vi "质控启动参数选择对话框.vi"(6 "CODCr":bool, 8 "CODMn":bool, 9 "总氮":bool, 10 "总磷":bool, 11 "氨氮":bool) -> (1 "取消启动":bool, 2 "确定启动":bool, 3 "启动模块":T1)   [LabVIEW 2016, in "质控单元.lvlib"]
uses:
  <vilib>/Utility/miscctls.llb/LVPointTypeDef.ctl
panel:
  in  "CODCr":bool
  in  "总氮":bool
  in  "确定":bool
  in  "CODMn":bool
  in  "总磷":bool
  in  "取消":bool
  in  "氨氮":bool
  # "请选择加标回收模块"
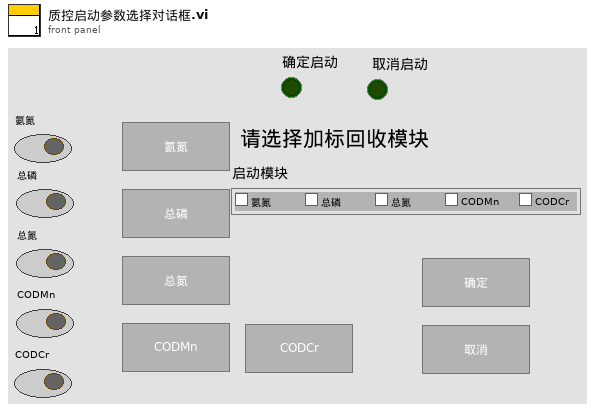
[diagram p1: front panel]
types:
  T1 = cluster{"氨氮":bool, "总磷":bool, "总氮":bool, "CODMn":bool, "CODCr":bool}
  T2 = typedef "LVPointTypeDef.ctl" = cluster{"Horizontal":i16, "Vertical":i16}
  T3 = enum8{"Enabled", "Disabled", "Disabled and Grayed Out"}
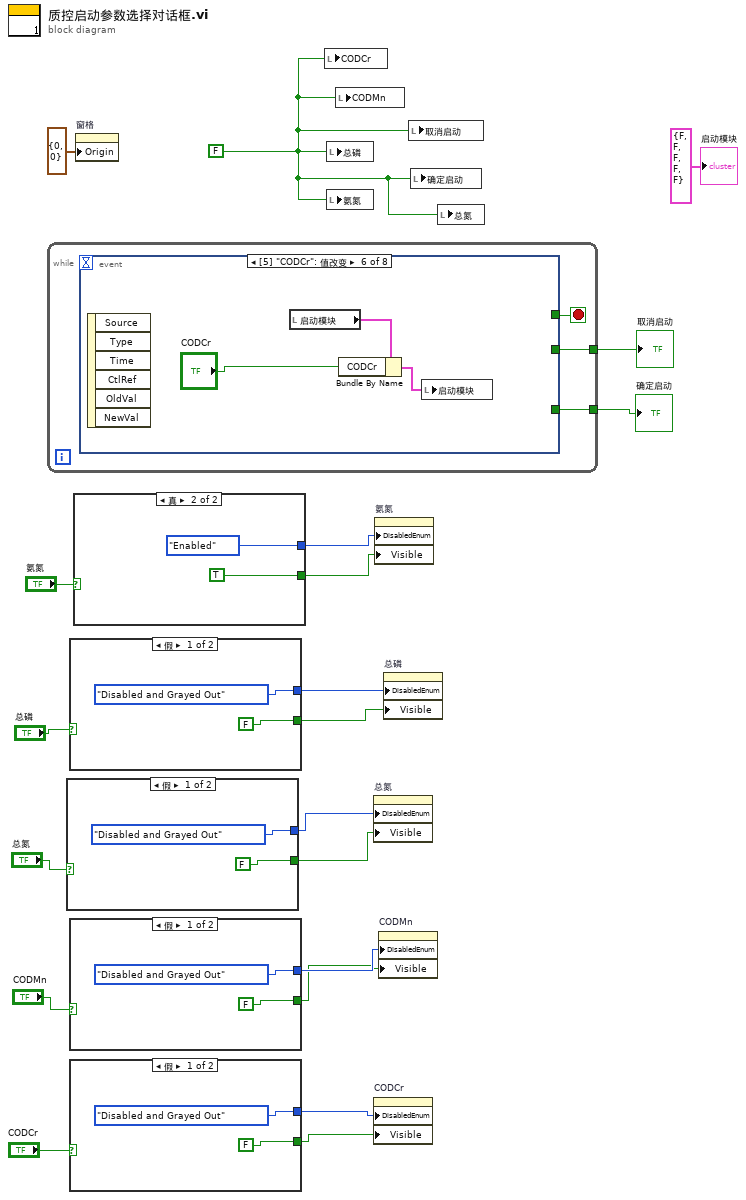
[diagram p0: block diagram]
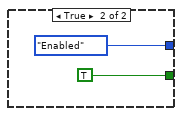
[diagram p2: hidden frame]
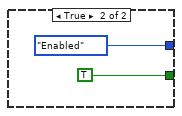
[diagram p3: hidden frame]
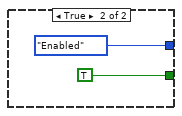
[diagram p4: hidden frame]
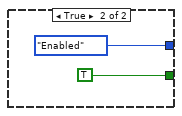
[diagram p5: hidden frame]
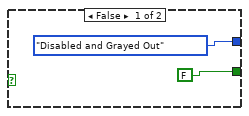
[diagram p6: hidden frame]
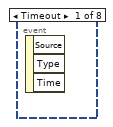
[diagram p7: hidden frame]
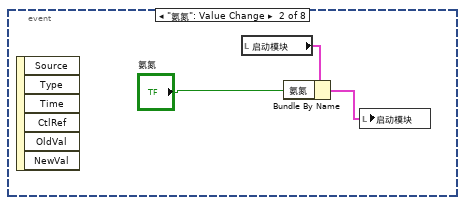
[diagram p8: hidden frame]
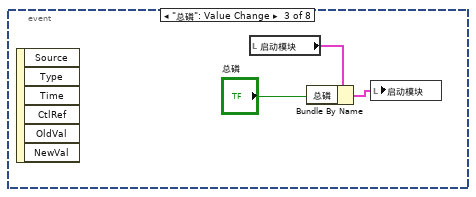
[diagram p9: hidden frame]
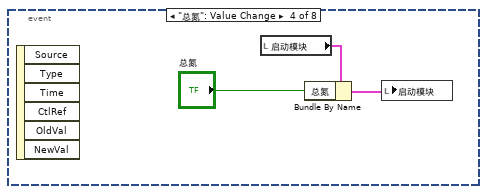
[diagram p10: hidden frame]
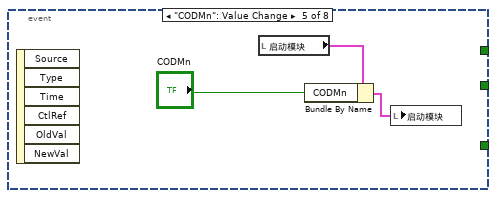
[diagram p11: hidden frame]
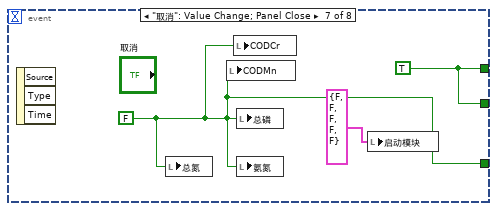
[diagram p12: hidden frame]
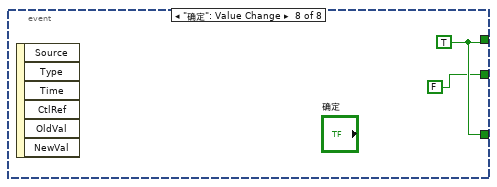
[diagram p13: hidden frame]
diagram:
  w5 = FALSE ("确定")
  n1 = while {
    tunnel: [w22] -> w20
    tunnel: [w21] -> w19
    stop <- w23 stop-if-true
    n2 = event shown="[5] \"CODCr\": 值改变" {
      selector: _ -> [_ _ _ _ _ _ _ _]
      dyn-events: _ -> [_ _ _ _ _ _ _ _]
      timeout: _ -> [_ _ _ _ _ _ _ _]
      tunnel: [_ _ _ _ _ _ w41 w43] -> w23
      tunnel: [_ _ _ _ _ _ w40 w43] -> w22
      tunnel: [_ _ _ _ _ _ w41 FALSE ("确定")] -> w21
      event Timeout {
        n3 = event-data() -> ()  [unwired: 1 in, 3 out]
      }
      event "氨氮": Value Change {
        n4 = event-data() -> ()  [unwired: 1 in, 6 out]
        n5 = local read "启动模块"() -> (w25:T1)
        n6 = Bundle By Name(cluster=w25, "氨氮"="氨氮") -> (w24:T1)
        n7 = local write "启动模块"(w24) -> ()
      }
      event "总磷": Value Change {
        n8 = event-data() -> ()  [unwired: 1 in, 6 out]
        n9 = local read "启动模块"() -> (w28:T1)
        n10 = Bundle By Name(cluster=w28, "总磷"="总磷") -> (w27:T1)
        n11 = local write "启动模块"(w27) -> ()
      }
      event "总氮": Value Change {
        n12 = event-data() -> ()  [unwired: 1 in, 6 out]
        n13 = local read "启动模块"() -> (w31:T1)
        n14 = Bundle By Name(cluster=w31, "总氮"="总氮") -> (w30:T1)
        n15 = local write "启动模块"(w30) -> ()
      }
      event "CODMn": Value Change {
        n16 = event-data() -> ()  [unwired: 1 in, 6 out]
        n17 = local read "启动模块"() -> (w34:T1)
        n18 = Bundle By Name(cluster=w34, "CODMn"="CODMn") -> (w33:T1)
        n19 = local write "启动模块"(w33) -> ()
      }
      event "CODCr": Value Change {
        n20 = event-data() -> ()  [unwired: 1 in, 6 out]
        n21 = local read "启动模块"() -> (w38:T1)
        n22 = Bundle By Name(cluster=w38, "CODCr"="CODCr") -> (w37:T1)
        n23 = local write "启动模块"(w37) -> ()
      }
      event "取消": Value Change; Panel Close {
        w40 = FALSE ("确定")
        w41 = TRUE ("确定")
        n24 = event-data() -> ()  [unwired: 1 in, 3 out]
        n25 = local write "总氮"(w40) -> ()
        n26 = local write "CODMn"(w40) -> ()
        n27 = local write "CODCr"(w40) -> ()
        n28 = local write "总磷"(w40) -> ()
        n29 = local write "氨氮"(w40) -> ()
        n30 = local write "启动模块"(T1 {"氨氮"=FALSE, "总磷"=FALSE, "总氮"=FALSE, "CODMn"=FALSE, "CODCr"=FALSE} ("启动模块")) -> ()
      }
      event "确定": Value Change {
        w43 = TRUE ("确定")
        n31 = event-data() -> ()  [unwired: 1 in, 6 out]
      }
    }
  }
  "确定启动" <- w20
  "取消启动" <- w19
  n32 = case shown="假" "总氮" {
    tunnel: [T3."Disabled and Grayed Out" ("禁用") T3."Enabled" ("禁用")] -> w10
    tunnel: [FALSE ("可见") TRUE ("可见")] -> w9
    frame False {
    }
    frame True {
    }
  }
  n33 = case shown="假" "总磷" {
    tunnel: [T3."Disabled and Grayed Out" ("禁用") T3."Enabled" ("禁用")] -> w12
    tunnel: [FALSE ("可见") TRUE ("可见")] -> w11
    frame False {
    }
    frame True {
    }
  }
  n34 = case shown="假" "CODMn" {
    tunnel: [T3."Disabled and Grayed Out" ("禁用") T3."Enabled" ("禁用")] -> w8
    tunnel: [FALSE ("可见") TRUE ("可见")] -> w7
    frame False {
    }
    frame True {
    }
  }
  n35 = case shown="假" "CODCr" {
    tunnel: [T3."Disabled and Grayed Out" ("禁用") T3."Enabled" ("禁用")] -> w2
    tunnel: [FALSE ("可见") TRUE ("可见")] -> w1
    frame False {
    }
    frame True {
    }
  }
  n36 = case shown="真" "氨氮" {
    tunnel: [T3."Disabled and Grayed Out" ("禁用") T3."Enabled" ("禁用")] -> w14
    tunnel: [FALSE ("可见") TRUE ("可见")] -> w13
    frame False {
    }
    frame True {
    }
  }
  n37 = property on="窗格" class="Pane"("Origin"=T2 {"Horizontal"=0, "Vertical"=0} ("原点")) -> ()  [unwired: 2 in, 2 out]
  n38 = local write "CODCr"(w5) -> ()
  n39 = local write "总磷"(w5) -> ()
  n40 = local write "氨氮"(w5) -> ()
  n41 = local write "CODMn"(w5) -> ()
  n42 = property on="总氮" class="Bool (严格)"("DisabledEnum"=w10, "Visible"=w9) -> ()  [unwired: 2 in, 2 out]
  n43 = property on="CODCr" class="Bool (严格)"("DisabledEnum"=w2, "Visible"=w1) -> ()  [unwired: 2 in, 2 out]
  n44 = property on="氨氮" class="Bool (严格)"("DisabledEnum"=w14, "Visible"=w13) -> ()  [unwired: 2 in, 2 out]
  n45 = property on="CODMn" class="Bool (严格)"("DisabledEnum"=w8, "Visible"=w7) -> ()  [unwired: 2 in, 2 out]
  n46 = property on="总磷" class="Bool (严格)"("DisabledEnum"=w12, "Visible"=w11) -> ()  [unwired: 2 in, 2 out]
  n47 = local write "取消启动"(w5) -> ()
  n48 = local write "确定启动"(w5) -> ()
  n49 = local write "总氮"(w5) -> ()
  "启动模块" <- T1 {"氨氮"=FALSE, "总磷"=FALSE, "总氮"=FALSE, "CODMn"=FALSE, "CODCr"=FALSE} ("启动模块")
